vi "Play WAV File.vi"() -> ()   [LabVIEW 2010]
uses:
  <vilib>/sound2/lvsound2.llb/Sampling Mode.ctl
  <vilib>/sound2/lvsound2.llb/Sound File Position.ctl
  <vilib>/sound2/lvsound2.llb/Sound File Info (path).vi
  <vilib>/sound2/lvsound2.llb/Sound File Read Open.vi
  <vilib>/sound2/lvsound2.llb/Sound File Read (DBL).vi
  <vilib>/sound2/lvsound2.llb/Sound Output Write (DBL).vi
panel:
  out "Max Amplitude Per Sample Chunk":dbl[](graph)=[0.000518798828125, 0.012969970703125, 0.037445068359375, 0.0289306640625, 0.065521240234375, 0.12841796875, 0.146484375, 0.8829345703125, 0.881744384765625, 0.560882568359375, 0.563812255859375, 0.879669189453125, 0.75799560546875, 0.878021240234375, 0.59857177734375, 0.836639404296875, 0.663360595703125, 0.509033203125, 0.450592041015625, 0.880615234375, 0.874298095703125, 0.6141357421875, 0.673187255859375, 0.87701416015625, 0.865966796875, 0.7266845703125, 0.63726806640625, 0.591766357421875, 0.65435791015625, 0.52972412109375, 0.562591552734375, 0.530548095703125, 0.14691162109375, 0.076690673828125, 0.087860107421875, 0.0596923828125, 0.037078857421875, 0.023162841796875, 0.023651123046875, 0.01434326171875, 0.007354736328125, 0.0037841796875, 0.002685546875, 0.00201416015625, 0.00146484375, 0.000732421875, 0.00054931640625, 0.000244140625, 0.000152587890625, 0.0001220703125, 9.1552734375e-05, 6.103515625e-05, 0.0001220703125, 0.00140380859375, 0.00335693359375, 0.005523681640625, 0.009979248046875, 0.01708984375, 0.018707275390625, 0.0269775390625, 0.03155517578125, 0.05560302734375, 0.075775146484375, 0.085845947265625, 0.091217041015625, 0.106048583984375, 0.107635498046875, 0.133636474609375, 0.166351318359375, 0.224884033203125, 0.207427978515625, 0.204864501953125, 0.181243896484375, 0.890869140625, 0.890869140625, 0.597381591796875, 0.77337646484375, 0.882110595703125, 0.707275390625, 0.5712890625, 0.68505859375, 0.890869140625, 0.890869140625, 0.806304931640625, 0.7310791015625, 0.88775634765625, 0.88262939453125, 0.848663330078125, 0.869293212890625, 0.890869140625, 0.890869140625, 0.80291748046875, 0.70941162109375, 0.5904541015625, 0.7640380859375, 0.517852783203125, 0.51171875, 0.431976318359375, 0.283233642578125, 0.087677001953125, 0.059356689453125, 0.0537109375, 0.046051025390625, 0.038238525390625, 0.031036376953125, 0.02825927734375, 0.0235595703125, 0.024566650390625, 0.02587890625, 0.025299072265625, 0.02459716796875, 0.019927978515625, 0.0, 0.0, 0.0, 0.0, 0.0, 0.0, 0.0, 0.0, 0.0, 0.0, 0.0, 0.0, 0.0, 0.0, 0.0, 0.0, 0.0, 0.0, 0.0, 0.0, 0.0, 0.0, 0.0, 0.014678955078125, 0.0391845703125, 0.110076904296875, 0.16986083984375, 0.890869140625, 0.890869140625, 0.633819580078125, 0.59033203125, 0.59710693359375, 0.097900390625, 0.1639404296875, 0.141021728515625, 0.87603759765625, 0.654998779296875, 0.5357666015625, 0.456024169921875, 0.433624267578125, 0.880035400390625, 0.8751220703125, 0.68310546875, 0.727142333984375, 0.890869140625, 0.78515625, 0.680267333984375, 0.610748291015625, 0.890869140625, 0.53082275390625, 0.492279052734375, 0.40081787109375, 0.322998046875, 0.1734619140625, 0.14306640625, 0.11077880859375, 0.19598388671875, 0.175262451171875, 0.19573974609375, 0.16473388671875, 0.1453857421875, 0.092498779296875, 0.043701171875, 0.055389404296875, 0.04583740234375, 0.01763916015625, 0.042724609375, 0.027496337890625, 0.024200439453125, 0.0211181640625]
  in  "Start Position (Samples)":i32
  out "Read Position (Samples)":i32=364000
  in  "Samples Per Read":i32=2000
  out "Sound File Info":waveform(dbl)[](graph)=[{"t0"=timestamp(1.0657596371882085 s since 1904-01-01), "dt"=2.2675736961451248e-05, "Y"=array[2000 elements]}, {"t0"=timestamp(1.0657596371882085 s since 1904-01-01), "dt"=2.2675736961451248e-05, "Y"=array[2000 elements]}]
  in  "stop":bool
  in  "WAV file location":path
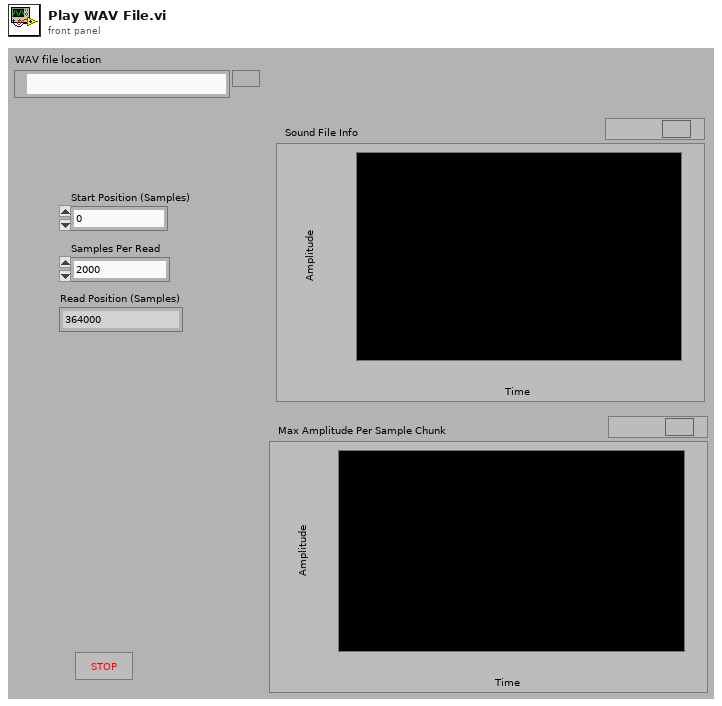
[diagram p1: front panel]
types:
  T1 = typedef "Sampling Mode.ctl" = i32
  T2 = typedef "Sound Data Format.ctl" = cluster{"sample rate (S/s)":dbl, "number of channels":i32, "bits per sample":i32}
  T3 = typedef "Sound File Refnum.ctl" = refnum<file>
  T4 = typedef "Sound Output Task ID.ctl" = u32
  T5 = typedef "Sound File Position.ctl" = u16
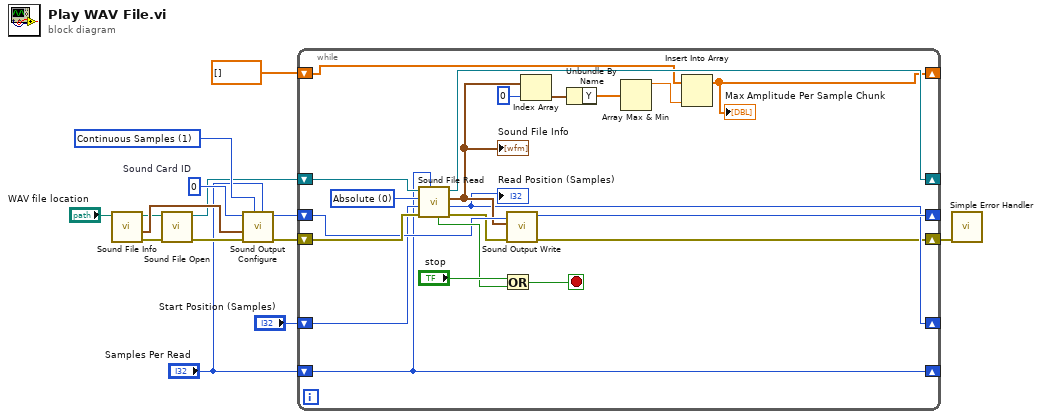
[diagram p0: block diagram]
diagram:
  w12 = T1 1 items=["Finite Samples", "Continuous Samples"] ("sample mode")
  w14 = u32 0  # Sound Card ID
  n1 = call-poly <vilib>:"Sound File Info.vi"("path"="WAV file location") -> ("error out"=w9:errorcluster, "sound format"=w13:T2, "path out"=w6:path)  [unwired: 7 in, 1 out]
  n2 = call-poly <vilib>:"Sound File Open.vi"("error in (no error)"=w9, "path"=w6) -> ("error out"=w8:errorcluster, "sound file refnum"=w10:T3)  [unwired: 8 in]
  n3 = call <vilib>:"Sound Output Configure.vi"("number of samples/ch"="Samples Per Read", "sample mode"=w12, "error in (no error)"=w8, "sound format"=w13, "device ID"=w14) -> ("error out"=w3:errorcluster, "task ID"=w11:T4)  [unwired: 5 in]
  n4 = while {
    shift-right: [w26] -> _
    shift-left: w11 -> [w29]
    shift-right: [w15] -> w1
    shift-left: w3 -> [w34]
    shift-right: [w30] -> _
    shift-left: w10 -> [w35]
    shift-right: [w20] -> _
    shift-left: "Samples Per Read" -> [w20]
    shift-right: [w16] -> _
    shift-left: "Start Position (Samples)" -> [w27]
    shift-right: [w19] -> _
    shift-left: dbl[] [] -> [w22]
    stop <- w21 stop-if-true
    w33 = T5 0 items=["Absolute"=0, "Relative"=2] ("position mode")
    n5 = call-poly <vilib>:"Sound File Read.vi"("number of samples/ch (-1: all)"=w20, "error in (no error)"=w34, "position offset"=w27, "position mode"=w33, "sound file refnum"=w35) -> ("error out"=w28:errorcluster, "offset"=w16:i32, "data"=w25:waveform(dbl)[], "sound file refnum out"=w30:T3, "end of file?"=w31:bool)  [unwired: 2 in]
    "Sound File Info" <- w25
    "Read Position (Samples)" <- w16
    n6 = Or(x="stop", y=w31) -> (x .or. y?=w21:bool)
    n7 = call-poly <vilib>:"Sound Output Write.vi"("error in (no error)"=w28, "data"=w25, "task ID"=w29) -> ("error out"=w15:errorcluster, "task ID out"=w26:T4)  [unwired: 7 in]
    n8 = Index Array(array=w25, index=0) -> (element=w23:waveform(dbl))
    n9 = Unbundle By Name(w23) -> ("Y"=w18:dbl[])
    n10 = Array Max & Min(array=w18) -> (max value=w17:dbl)  [unwired: 3 out]
    n11 = Insert Into Array(array=w22, new element=w17) -> (w19:dbl[])  [unwired: 1 in]
    "Max Amplitude Per Sample Chunk" <- w19
  }
  n12 = call <vilib>:"Simple Error Handler.vi"("error in (no error)"=w1) -> ()  [unwired: 4 in, 5 out]
